vi "Firmware Wizard.vi"() -> ()   [LabVIEW 2011, in "LVH-LINX.lvlib"]
doc: "Wizard for uploading firmware to LINX devices."
uses:
  LVH-LINX.lvlib
  Type Defs/Device Family.ctl
  Type Defs/Deploy Firmware State.ctl
  <vilib>/LabVIEW Hacker/LVH-Toolbox/Common/LVH-Common.lvlib
panel:
  in  "Device Family Enum":T1
  out "Error Out":errorcluster
  in  "Error In":errorcluster
  out "Tab Control":T2(tab)
  in  "Settings Button":bool
  out "Device Image":picture
  in  "Device Help":bool
  in  "Firmware Program Interface":u16(ring) items=["Serial / USB"]
  in  "Device Type":u16(ring) items=["chipKIT Uno32", "chipKIT uC32", "chipKIT Max32", "chipKIT DP32"]
  in  "Device Family":u16(ring) items=["National Instruments", "Digilent", "Arduino"]
  in  "Device Cancel":bool
  in  "Device Next":bool
  in  "Device Noticiation":string
  in  "Config Message":string
  in  "Int Help":bool
  in  "Int Previous":bool
  in  "Int Cancel":bool
  in  "Int Next":bool
  out "Interface Config":enum32{"N/A", "Serial / USB", "USB", "TCP"}(tab)
  in  "COM Port":refnum<visa-resource-name>
  in  "Firmware Description":string
  in  "FWV Help":bool
  in  "FWV Cancel":bool
  in  "FWV Next":bool
  in  "FWV Previous":bool
  in  "Firmware Version":u16(ring) items=["LINX -  Serial / USB", "LINX -  Serial / USB [Debug] "]
  in  "Deploy  Progress Bar":u8(slide) scale=0.0..100.0
  in  "LINX Forum Link":string="www.labviewhacker.com/forums/linx"
  in  "LINX Landing Page Link":string="www.labviewhacker.com/linx"
  in  "Summary Launch Example":bool
  in  "Summary Text":string
  in  "Summary Next":bool
  in  "Summary Help":bool
  # "Uploading Firmware..."
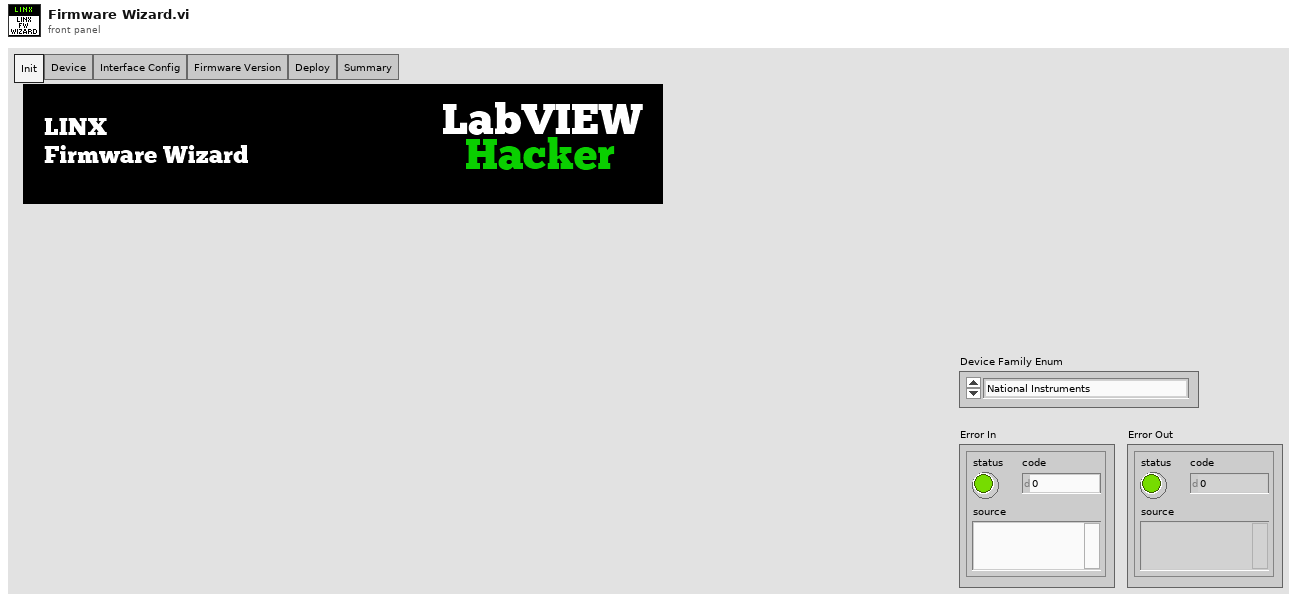
[diagram p1: front panel]
types:
  T1 = typedef "LVH-LINX.lvlib/Device Family.ctl" = enum8{"National Instruments", "Digilent", "Arduino"}
  T2 = enum32{"Init", "Device", "Interface Config", "Firmware Version", "Deploy", "Summary"}
  T3 = typedef "LVH-LINX.lvlib/Deploy Firmware State.ctl" = enum32{"Init", "Device", "Interface Config", "Firmware Version", "Deploy", "Summary"}
  T4 = enum16{"Left Button", "Center Button", "Right Button", "Window Close"}
  T5 = enum32{"invalid app kind", "Development System", "Run Time System", "Student Edition", "Embedded LabVIEW", "Evaluation", "Custom"}
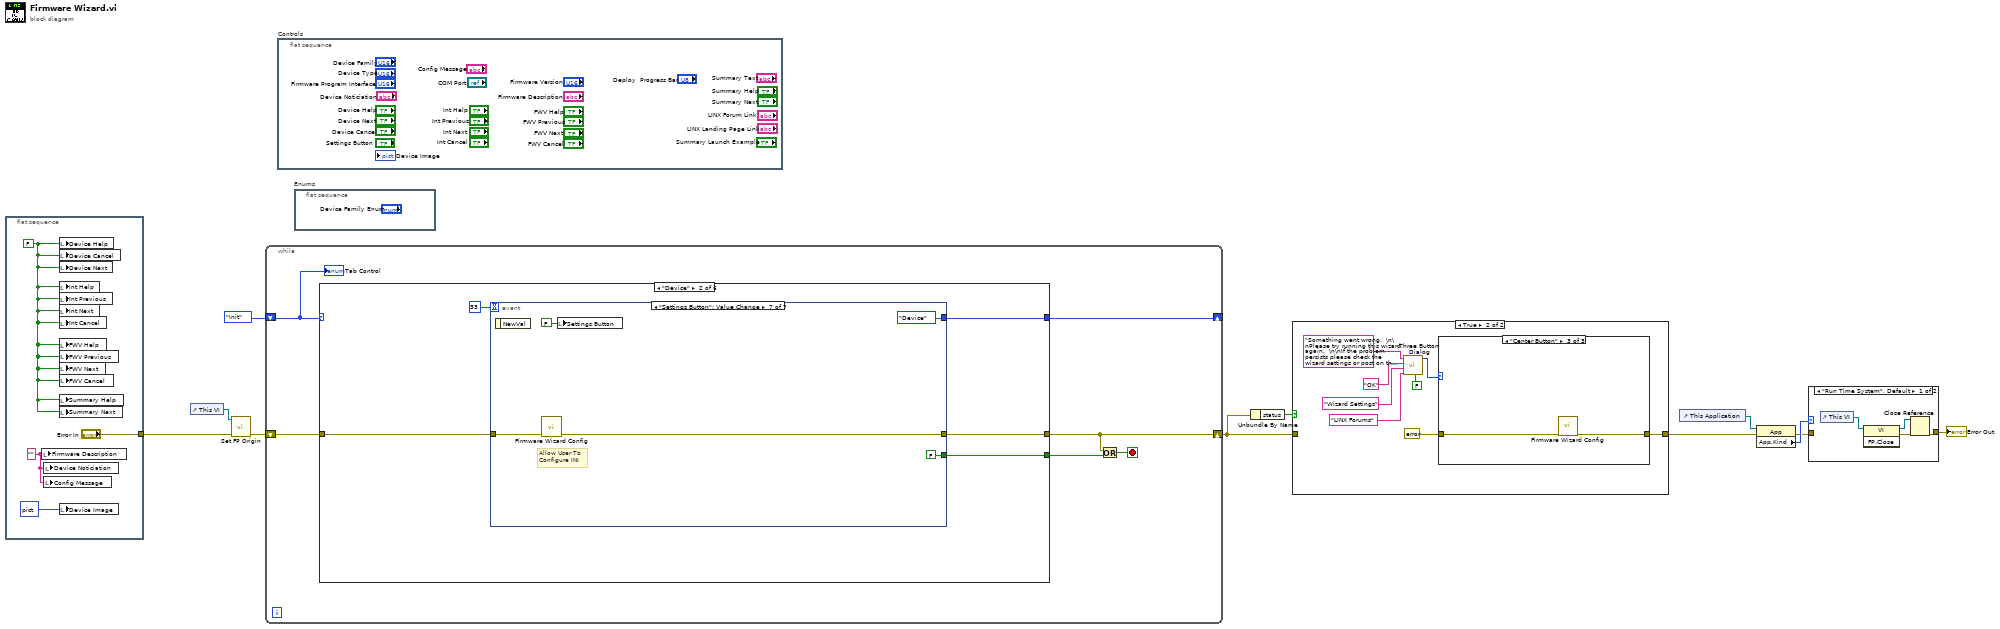
[diagram p0: block diagram]
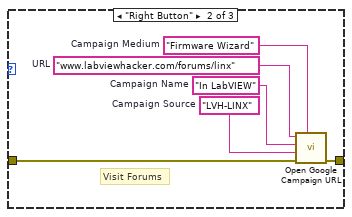
[diagram p4: hidden frame]
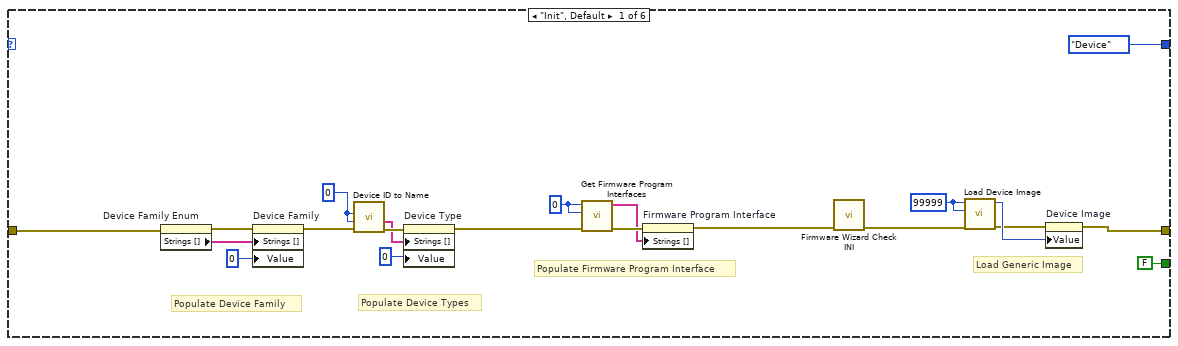
[diagram p6: hidden frame]
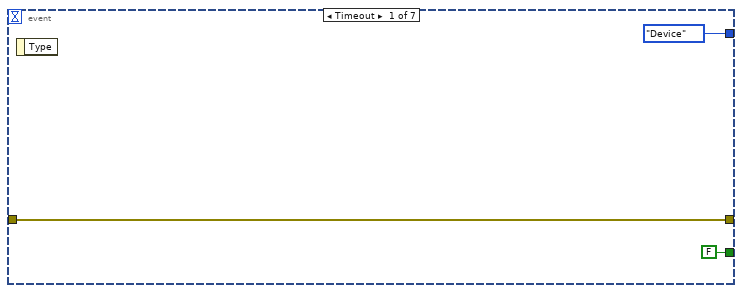
[diagram p7: hidden frame]
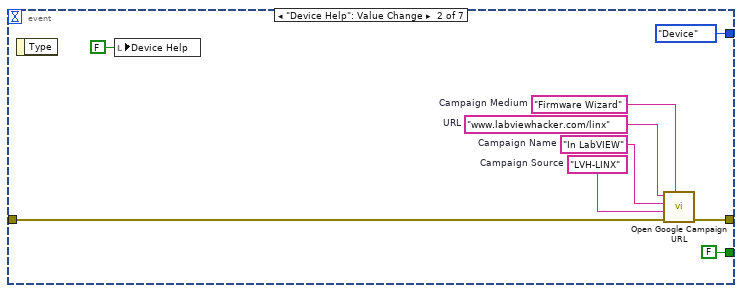
[diagram p8: hidden frame]
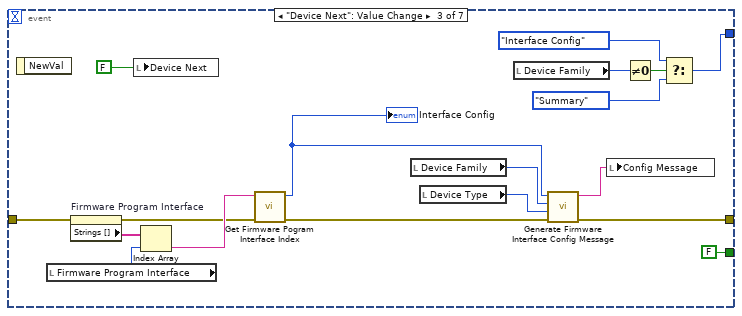
[diagram p9: hidden frame]
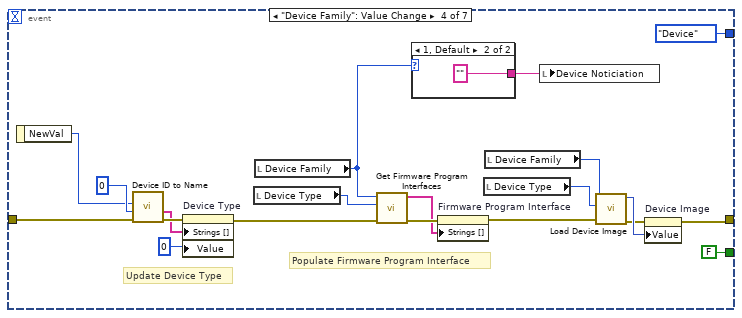
[diagram p10: hidden frame]
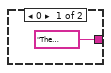
[diagram p11: hidden frame]
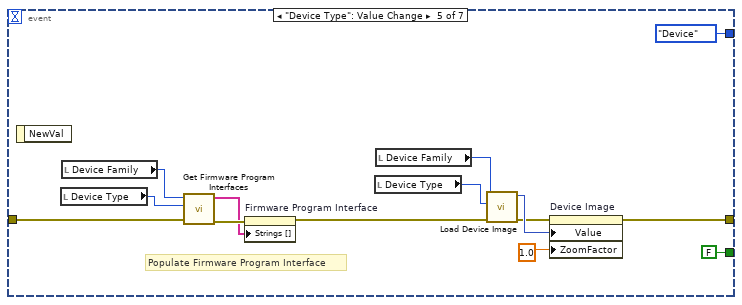
[diagram p12: hidden frame]
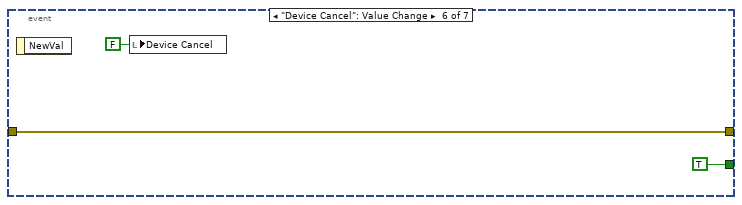
[diagram p13: hidden frame]
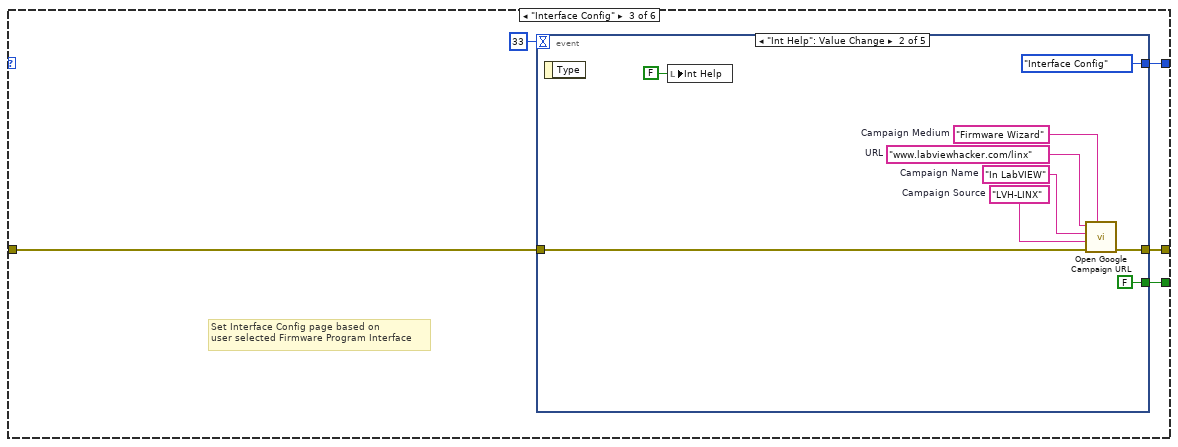
[diagram p14: hidden frame]
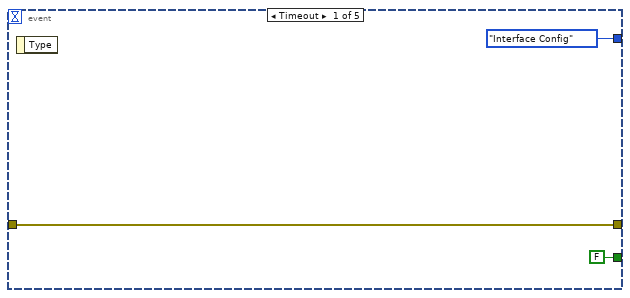
[diagram p15: hidden frame]
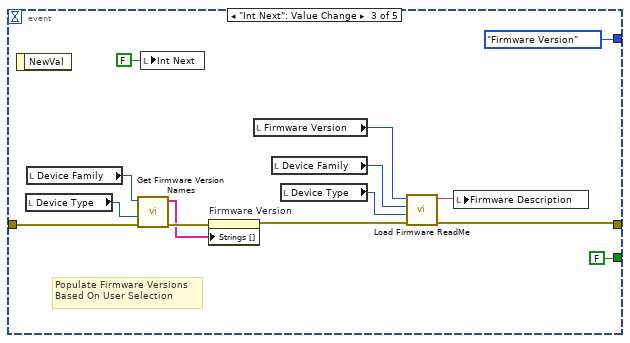
[diagram p16: hidden frame]
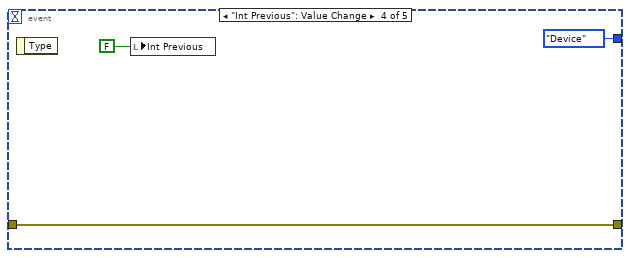
[diagram p17: hidden frame]
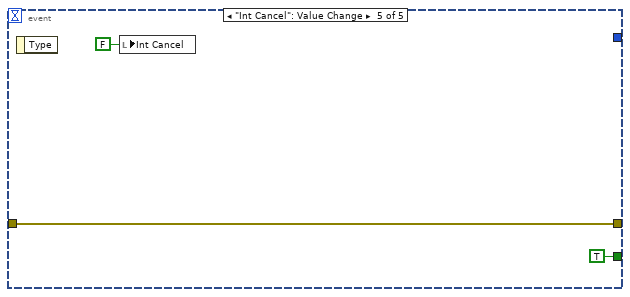
[diagram p18: hidden frame]
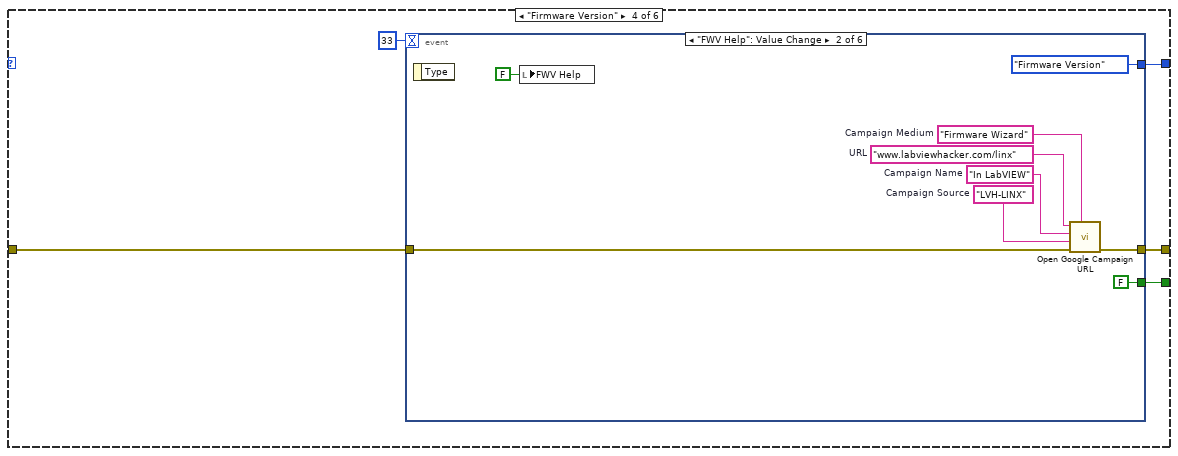
[diagram p19: hidden frame]
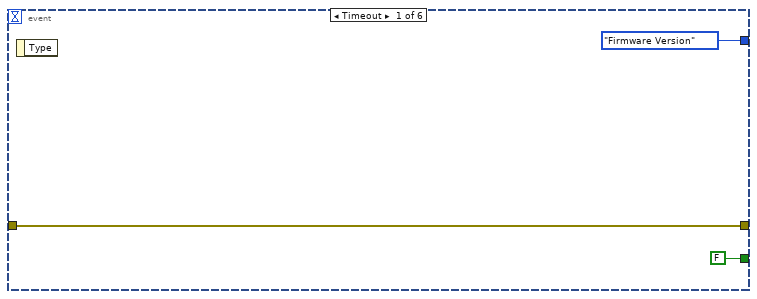
[diagram p20: hidden frame]
diagram:
  n1 = flat-sequence {
    tunnel: ["Error In"] -> w9
    frame #0 {
      w12 = "" ("Firmware Description")
      w14 = FALSE ("Cancel")
      n2 = local write "Firmware Description"(w12) -> ()
      n3 = local write "Device Noticiation"(w12) -> ()
      n4 = local write "Config Message"(w12) -> ()
      n5 = local write "Device Help"(w14) -> ()
      n6 = local write "Device Cancel"(w14) -> ()
      n7 = local write "Device Next"(w14) -> ()
      n8 = local write "Int Help"(w14) -> ()
      n9 = local write "Int Previous"(w14) -> ()
      n10 = local write "Int Next"(w14) -> ()
      n11 = local write "Int Cancel"(w14) -> ()
      n12 = local write "FWV Help"(w14) -> ()
      n13 = local write "FWV Previous"(w14) -> ()
      n14 = local write "FWV Next"(w14) -> ()
      n15 = local write "FWV Cancel"(w14) -> ()
      n16 = local write "Summary Help"(w14) -> ()
      n17 = local write "Summary Next"(w14) -> ()
      n18 = local write "Device Image"(picture data[5B] ("2D Picture")) -> ()
    }
  }
  n19 = control-ref of="This VI"() -> (w10:refnum<vi>)
  n20 = call <vilib>:"Set FP Origin.vi"("Error In"=w9, "VI Ref"=w10) -> ("Error Out"=w8:errorcluster)  [unwired: 9 in]
  n21 = while {
    shift-right: [w19] -> _
    shift-left: Deploy_Firmware_State."Init" ("Deploy Firmware State") -> [w21]
    shift-right: [w18] -> w1
    shift-left: w8 -> [w20]
    stop <- w17 stop-if-true
    n22 = case shown="\"Device\"" w21 {
      tunnel: [w25 w46 w125 w163 w201 w213] -> w18
      tunnel: w20 -> [w29 w45 w122 w162 w202 w209]
      tunnel: [Deploy_Firmware_State."Device" ("Deploy Firmware State") w44 w126 w160 Deploy_Firmware_State."Summary" ("Deploy Firmware State") w211] -> w19
      tunnel: [FALSE w43 w123 w159 FALSE w210] -> w16
      frame "Init", Default {
        w24 = u32 99999 ("Device Family")
        w30 = u32 0 ("Device Family")
        w36 = u32 0 ("Device Family")
        # "Load Generic Image"
        # "Populate Firmware Program Interface"
        # "Populate Device Types"
        # "Populate Device Family"
        n23 = property on="Device Family Enum" class="Enum (strict)"(error in=w29) -> (error out=w41:errorcluster, "Strings []"=w40:string[])  [unwired: 1 in, 1 out]
        n24 = property on="Device Family" class="Ring (strict)"(error in=w41, "Strings []"=w40, "Value"=u16 0 ("Device Family")) -> (error out=w38:errorcluster)  [unwired: 1 in, 1 out]
        n25 = call "Device ID to Name.vi"("Error In"=w38, "Device ID"=w36, "Device Family"=w36) -> ("Error Out"=w37:errorcluster, "Devices In Family"=w35:string[])  [unwired: 5 in, 2 out]
        n26 = property on="Device Type" class="Ring (strict)"(error in=w37, "Strings []"=w35, "Value"=u16 0 ("Device Family")) -> (error out=w31:errorcluster)  [unwired: 1 in, 1 out]
        n27 = call "Get Firmware Program Interfaces.vi"("Error In"=w31, "Device ID"=w30, "Device Family"=w30) -> ("Error Out"=w33:errorcluster, "Firmware Program Interfaces"=w32:string[])  [unwired: 7 in]
        n28 = property on="Firmware Program Interface" class="Ring (strict)"(error in=w33, "Strings []"=w32) -> (error out=w23:errorcluster)  [unwired: 1 in, 1 out]
        n29 = call "Firmware Wizard Check INI.vi"("Error In"=w23) -> ("Error Out"=w22:errorcluster)  [unwired: 10 in]
        n30 = call "Load Device Image.vi"("Error In"=w22, "Device Type"=w24, "Device Family"=w24) -> ("Error Out"=w26:errorcluster, "Device Image"=w27:picture)  [unwired: 7 in]
        n31 = property on="Device Image" class="Pict"(error in=w26, "Value"=w27) -> (error out=w25:errorcluster)  [unwired: 1 in, 1 out]
      }
      frame "Device" {
        n32 = event shown="[6] \"Settings Button\": Value Change" {
          selector: _ -> [_ _ _ _ _ _ _]
          dyn-events: _ -> [_ _ _ _ _ _ _]
          timeout: 33 -> [_ _ _ _ _ _ _]
          tunnel: [w50 w53 w68 w80 w100 w115 w118] -> w46
          tunnel: w45 -> [w50 w52 w62 w93 w113 w115 w119]
          tunnel: [Deploy_Firmware_State."Device" ("Deploy Firmware State") Deploy_Firmware_State."Device" ("Deploy Firmware State") w71 Deploy_Firmware_State."Device" ("Deploy Firmware State") Deploy_Firmware_State."Device" ("Deploy Firmware State") _ Deploy_Firmware_State."Device" ("Deploy Firmware State")] -> w44
          tunnel: [FALSE FALSE FALSE FALSE FALSE TRUE FALSE] -> w43
          event Timeout {
            n33 = event-data() -> ()  [unwired: 1 in, 1 out]
          }
          event "Device Help": Value Change {
            w51 = "LVH-LINX"  # Campaign Source
            w54 = "In LabVIEW"  # Campaign Name
            w55 = "Firmware Wizard"  # Campaign Medium
            w56 = "www.labviewhacker.com/linx"  # URL
            n34 = event-data() -> ()  [unwired: 1 in, 1 out]
            n35 = local write "Device Help"(FALSE ("Device Help")) -> ()
            n36 = call <vilib>:"Open Google Campaign URL.vi"("Campaign Medium"=w55, "Error In"=w52, "Campaign Source"=w51, "Campaign Name"=w54, "URL"=w56) -> ("Error Out"=w53:errorcluster)  [unwired: 5 in, 1 out]
          }
          event "Device Next": Value Change {
            n37 = event-data() -> ()  [unwired: 1 in, 1 out]
            n38 = local read "Firmware Program Interface"() -> (w63:u16)
            n39 = property on="Firmware Program Interface" class="Ring (strict)"(error in=w62) -> (error out=w64:errorcluster, "Strings []"=w66:string[])  [unwired: 1 in, 1 out]
            n40 = local write "Device Next"(FALSE ("Next")) -> ()
            n41 = Index Array(array=w66, index=w63) -> (element=w65:string)
            n42 = call "Get Firmware Pogram Interface Index.vi"("Error In"=w64, "Firmware Program Interface"=w65) -> ("Error Out"=w61:errorcluster, "Interface Index"=w60:i32)  [unwired: 8 in]
            "Interface Config" <- w60
            n43 = local read "Device Family"() -> (w70:u16)
            n44 = local read "Device Type"() -> (w67:u16)
            n45 = local read "Device Family"() -> (w74:u16)
            n46 = call "Generate Firmware Interface Config Message.vi"("Error In"=w61, "Device Type"=w67, "Device Family"=w70, "Firmware Program Interface"=w60) -> ("Error Out"=w68:errorcluster, "Config Message"=w69:string)  [unwired: 6 in]
            n47 = local write "Config Message"(w69) -> ()
            n48 = Not Equal To 0?(x=w74) -> (x != 0?=w75:bool)
            n49 = Select(t=Deploy_Firmware_State."Interface Config" ("Deploy Firmware State"), s=w75, f=Deploy_Firmware_State."Summary" ("Deploy Firmware State")) -> (s? t:f=w71:T3)
          }
          event "Device Family": Value Change {
            # "Populate Firmware Program Interface"
            # "Update Device Type"
            n50 = event-data() -> ("NewVal"=w92:u16)  [unwired: 1 in]
            n51 = call "Device ID to Name.vi"("Error In"=w93, "Device ID"=u32 0 ("Device Family"), "Device Family"=w92) -> ("Error Out"=w97:errorcluster, "Devices In Family"=w95:string[])  [unwired: 5 in, 2 out]
            n52 = property on="Device Type" class="Ring (strict)"(error in=w97, "Strings []"=w95, "Value"=u16 0 ("Device Family")) -> (error out=w87:errorcluster)  [unwired: 1 in, 1 out]
            n53 = local read "Device Type"() -> (w88:u16)
            n54 = local read "Device Family"() -> (w79:u16)
            n55 = call "Get Firmware Program Interfaces.vi"("Error In"=w87, "Device ID"=w88, "Device Family"=w79) -> ("Error Out"=w90:errorcluster, "Firmware Program Interfaces"=w89:string[])  [unwired: 7 in]
            n56 = case shown="1, Default" w79 {
              tunnel: ["The National Instruments devices that support LINX do not require firmware updates." ("Device Noticiation") "" ("Device Noticiation")] -> w78
              frame 0 {
              }
              frame 1, Default {
              }
            }
            n57 = property on="Firmware Program Interface" class="Ring (strict)"(error in=w90, "Strings []"=w89) -> (error out=w81:errorcluster)  [unwired: 1 in, 1 out]
            n58 = local read "Device Type"() -> (w85:u16)
            n59 = local read "Device Family"() -> (w84:u16)
            n60 = local write "Device Noticiation"(w78) -> ()
            n61 = call "Load Device Image.vi"("Error In"=w81, "Device Type"=w85, "Device Family"=w84) -> ("Error Out"=w82:errorcluster, "Device Image"=w83:picture)  [unwired: 7 in]
            n62 = property on="Device Image" class="Pict"(error in=w82, "Value"=w83) -> (error out=w80:errorcluster)  [unwired: 1 in, 1 out]
          }
          event "Device Type": Value Change {
            # "Populate Firmware Program Interface"
            n63 = event-data() -> ()  [unwired: 1 in, 1 out]
            n64 = local read "Device Type"() -> (w109:u16)
            n65 = local read "Device Family"() -> (w108:u16)
            n66 = call "Get Firmware Program Interfaces.vi"("Error In"=w113, "Device ID"=w109, "Device Family"=w108) -> ("Error Out"=w112:errorcluster, "Firmware Program Interfaces"=w111:string[])  [unwired: 7 in]
            n67 = property on="Firmware Program Interface" class="Ring (strict)"(error in=w112, "Strings []"=w111) -> (error out=w106:errorcluster)  [unwired: 1 in, 1 out]
            n68 = local read "Device Type"() -> (w105:u16)
            n69 = local read "Device Family"() -> (w104:u16)
            n70 = call "Load Device Image.vi"("Error In"=w106, "Device Type"=w105, "Device Family"=w104) -> ("Error Out"=w101:errorcluster, "Device Image"=w103:picture)  [unwired: 7 in]
            n71 = property on="Device Image" class="Pict"(error in=w101, "Value"=w103, "ZoomFactor"=sgl 1.0 ("Zoom Factor")) -> (error out=w100:errorcluster)  [unwired: 1 in, 1 out]
          }
          event "Device Cancel": Value Change {
            n72 = event-data() -> ()  [unwired: 1 in, 1 out]
            n73 = local write "Device Cancel"(FALSE ("Device Cancel")) -> ()
          }
          event "Settings Button": Value Change {
            # "Allow User To \nConfigure INI"
            n74 = event-data() -> ()  [unwired: 1 in, 1 out]
            n75 = call "Firmware Wizard Config.vi"("Error In"=w119) -> ("Error Out"=w118:errorcluster)  [unwired: 10 in]
            n76 = local write "Settings Button"(FALSE ("Settings Button")) -> ()
          }
        }
      }
      frame "Interface Config" {
        # "Set Interface Config page based on \nuser selected Firmware Program Interface"
        n77 = event shown="[1] \"Int Help\": Value Change" {
          selector: _ -> [_ _ _ _ _]
          dyn-events: _ -> [_ _ _ _ _]
          timeout: 33 -> [_ _ _ _ _]
          tunnel: [Deploy_Firmware_State."Interface Config" ("Deploy Firmware State") Deploy_Firmware_State."Interface Config" ("Deploy Firmware State") Deploy_Firmware_State."Firmware Version" ("Deploy Firmware State") Deploy_Firmware_State."Device" ("Deploy Firmware State") _] -> w126
          tunnel: [w128 w130 w139 w155 w156] -> w125
          tunnel: w122 -> [w128 w131 w152 w155 w156]
          tunnel: [FALSE FALSE FALSE _ TRUE] -> w123
          event Timeout {
            n78 = event-data() -> ()  [unwired: 1 in, 1 out]
          }
          event "Int Help": Value Change {
            w132 = "LVH-LINX"  # Campaign Source
            w133 = "In LabVIEW"  # Campaign Name
            w134 = "Firmware Wizard"  # Campaign Medium
            w135 = "www.labviewhacker.com/linx"  # URL
            n79 = event-data() -> ()  [unwired: 1 in, 1 out]
            n80 = local write "Int Help"(FALSE ("Int Help")) -> ()
            n81 = call <vilib>:"Open Google Campaign URL.vi"("Campaign Medium"=w134, "Error In"=w131, "Campaign Source"=w132, "Campaign Name"=w133, "URL"=w135) -> ("Error Out"=w130:errorcluster)  [unwired: 5 in, 1 out]
          }
          event "Int Next": Value Change {
            # "Populate Firmware Versions\nBased On User Selection"
            n82 = event-data() -> ()  [unwired: 1 in, 1 out]
            n83 = local read "Device Type"() -> (w149:u16)
            n84 = local read "Device Family"() -> (w148:u16)
            n85 = call "Get Firmware Version Names.vi"("Error In"=w152, "Device ID"=w149, "Device Family"=w148) -> ("Error Out"=w151:errorcluster, "Firmware Version Names"=w150:string[])  [unwired: 6 in, 1 out]
            n86 = local write "Int Next"(FALSE ("Int Next")) -> ()
            n87 = property on="Firmware Version" class="Ring (strict)"(error in=w151, "Strings []"=w150) -> (error out=w140:errorcluster)  [unwired: 1 in, 1 out]
            n88 = local read "Firmware Version"() -> (w142:u16)
            n89 = local read "Device Family"() -> (w144:u16)
            n90 = local read "Device Type"() -> (w143:u16)
            n91 = call "Load Firmware ReadMe.vi"("Error In"=w140, "Device Family"=w143, "Device Type"=w144, "Firmware Version"=w142) -> ("Error Out"=w139:errorcluster, "Firmware ReadMe"=w141:string)  [unwired: 6 in]
            n92 = local write "Firmware Description"(w141) -> ()
          }
          event "Int Previous": Value Change {
            n93 = event-data() -> ()  [unwired: 1 in, 1 out]
            n94 = local write "Int Previous"(FALSE ("Previous")) -> ()
          }
          event "Int Cancel": Value Change {
            n95 = event-data() -> ()  [unwired: 1 in, 1 out]
            n96 = local write "Int Cancel"(FALSE ("Int Cancel")) -> ()
          }
        }
      }
      frame "Firmware Version" {
        n97 = event shown="[1] \"FWV Help\": Value Change" {
          selector: _ -> [_ _ _ _ _ _]
          dyn-events: _ -> [_ _ _ _ _ _]
          timeout: 33 -> [_ _ _ _ _ _]
          tunnel: [w166 w168 w178 w182 w186 w192] -> w163
          tunnel: w162 -> [w166 w167 w178 w182 w186 w193]
          tunnel: [Deploy_Firmware_State."Firmware Version" ("Deploy Firmware State") Deploy_Firmware_State."Firmware Version" ("Deploy Firmware State") Deploy_Firmware_State."Interface Config" ("Deploy Firmware State") Deploy_Firmware_State."Deploy" ("Deploy Firmware State") Deploy_Firmware_State."Init" ("Deploy Firmware State") Deploy_Firmware_State."Firmware Version" ("Deploy Firmware State")] -> w160
          tunnel: [FALSE FALSE FALSE FALSE TRUE FALSE] -> w159
          event Timeout {
            n98 = event-data() -> ()  [unwired: 1 in, 1 out]
          }
          event "FWV Help": Value Change {
            w169 = "LVH-LINX"  # Campaign Source
            w170 = "In LabVIEW"  # Campaign Name
            w171 = "Firmware Wizard"  # Campaign Medium
            w172 = "www.labviewhacker.com/linx"  # URL
            n99 = event-data() -> ()  [unwired: 1 in, 1 out]
            n100 = local write "FWV Help"(FALSE ("FWV Help")) -> ()
            n101 = call <vilib>:"Open Google Campaign URL.vi"("Campaign Medium"=w171, "Error In"=w167, "Campaign Source"=w169, "Campaign Name"=w170, "URL"=w172) -> ("Error Out"=w168:errorcluster)  [unwired: 5 in, 1 out]
          }
          event "FWV Previous": Value Change {
            n102 = event-data() -> ()  [unwired: 1 in, 1 out]
            n103 = local write "FWV Previous"(FALSE ("FWV Previous")) -> ()
          }
          event "FWV Next": Value Change {
            n104 = event-data() -> ()  [unwired: 1 in, 1 out]
            n105 = local write "FWV Next"(FALSE ("FWV Previous")) -> ()
          }
          event "FWV Cancel": Value Change {
            n106 = event-data() -> ()  [unwired: 1 in, 1 out]
            n107 = local write "FWV Cancel"(FALSE ("FWV Previous")) -> ()
          }
          event "Firmware Version": Value Change {
            n108 = event-data() -> ()  [unwired: 1 in, 1 out]
            n109 = local read "Firmware Version"() -> (w189:u16)
            n110 = local read "Device Family"() -> (w191:u16)
            n111 = local read "Device Type"() -> (w190:u16)
            n112 = call "Load Firmware ReadMe.vi"("Error In"=w193, "Device Family"=w190, "Device Type"=w191, "Firmware Version"=w189) -> ("Error Out"=w192:errorcluster, "Firmware ReadMe"=w188:string)  [unwired: 6 in]
            n113 = local write "Firmware Description"(w188) -> ()
          }
        }
      }
      frame "Deploy" {
        n114 = control-ref of="Deploy  Progress Bar"() -> (w196:refnum<vi>)
        n115 = local read "Firmware Version"() -> (w200:u16)
        n116 = local read "Device Family"() -> (w198:u16)
        n117 = local read "Device Type"() -> (w199:u16)
        n118 = local read "COM Port"() -> (w197:refnum<visa-resource-name>)
        n119 = call "Upload Firmware.vi"("Progress Bar"=w196, "COM Port"=w197, "Error In"=w202, "Firmware Version"=w200, "Device ID"=w199, "Device Family"=w198) -> ("Error Out"=w201:errorcluster)  [unwired: 5 in]
      }
      frame "Summary" {
        n120 = local read "Device Family"() -> (w207:u16)
        n121 = local read "Device Type"() -> (w206:u16)
        n122 = call "Generate Firmware Wizard Summary Message.vi"("Error In"=w209, "Device ID"=w206, "Device Family"=w207) -> ("Error Out"=w208:errorcluster, "Summary"=w205:string)  [unwired: 7 in]
        n123 = local write "Summary Text"(w205) -> ()
        n124 = event shown="[3] \"Summary Help\": Value Change" {
          selector: _ -> [_ _ _ _ _ _]
          dyn-events: _ -> [_ _ _ _ _ _]
          timeout: 33 -> [_ _ _ _ _ _]
          tunnel: [w216 w223 w230 w238 w240 w245] -> w213
          tunnel: w208 -> [w216 w222 w229 w237 w240 w245]
          tunnel: [Deploy_Firmware_State."Summary" ("Deploy Firmware State") Deploy_Firmware_State."Summary" ("Deploy Firmware State") Deploy_Firmware_State."Summary" ("Deploy Firmware State") Deploy_Firmware_State."Summary" ("Deploy Firmware State") Deploy_Firmware_State."Summary" ("Deploy Firmware State") Deploy_Firmware_State."Init" ("Deploy Firmware State")] -> w211
          tunnel: [FALSE _ _ _ _ TRUE] -> w210
          event Timeout {
            n125 = event-data() -> ()  [unwired: 1 in, 1 out]
          }
          event "LINX Forum Link": Mouse Down {
            w218 = "LVH-LINX"  # Campaign Source
            w219 = "In LabVIEW"  # Campaign Name
            w220 = "Firmware Wizard"  # Campaign Medium
            w221 = "www.labviewhacker.com/forum/linx"  # URL
            n126 = event-data() -> ()  [unwired: 1 in, 7 out]
            n127 = call <vilib>:"Open Google Campaign URL.vi"("Campaign Medium"=w220, "Error In"=w222, "Campaign Source"=w218, "Campaign Name"=w219, "URL"=w221) -> ("Error Out"=w223:errorcluster)  [unwired: 5 in, 1 out]
          }
          event "LINX Landing Page Link": Mouse Down {
            w225 = "LVH-LINX"  # Campaign Source
            w226 = "In LabVIEW"  # Campaign Name
            w227 = "Firmware Wizard"  # Campaign Medium
            w228 = "www.labviewhacker.com/linx"  # URL
            n128 = event-data() -> ()  [unwired: 1 in, 7 out]
            n129 = call <vilib>:"Open Google Campaign URL.vi"("Campaign Medium"=w227, "Error In"=w229, "Campaign Source"=w225, "Campaign Name"=w226, "URL"=w228) -> ("Error Out"=w230:errorcluster)  [unwired: 5 in, 1 out]
          }
          event "Summary Help": Value Change {
            w233 = "LVH-LINX"  # Campaign Source
            w234 = "In LabVIEW"  # Campaign Name
            w235 = "Firmware Wizard"  # Campaign Medium
            w236 = "www.labviewhacker.com/linx"  # URL
            n130 = event-data() -> ()  [unwired: 1 in, 1 out]
            n131 = local write "Summary Help"(FALSE ("Summary Help")) -> ()
            n132 = call <vilib>:"Open Google Campaign URL.vi"("Campaign Medium"=w235, "Error In"=w237, "Campaign Source"=w233, "Campaign Name"=w234, "URL"=w236) -> ("Error Out"=w238:errorcluster)  [unwired: 5 in, 1 out]
          }
          event "Summary Launch Example": Value Change {
            n133 = event-data() -> ()  [unwired: 1 in, 1 out]
            n134 = local write "Summary Launch Example"(FALSE ("Summary Launch Example")) -> ()
            n135 = One Button Dialog(message="Feature Not Yet Implemented") -> ()  [unwired: 1 in, 1 out]
          }
          event "Summary Next": Value Change {
            n136 = event-data() -> ()  [unwired: 1 in, 1 out]
            n137 = local write "Summary Next"(FALSE ("FWV Previous")) -> ()
          }
        }
      }
    }
    n138 = Or(x=w18, y=w16) -> (x .or. y?=w17:bool)
    "Tab Control" <- w21
  }
  n139 = flat-sequence "Controls" {
    frame #0 {
    }
  }
  n140 = flat-sequence "Enums" {
    frame #0 {
    }
  }
  n141 = Unbundle By Name(w1) -> ("status"=w3:bool)
  n142 = case shown="True" w3 {
    tunnel: [w247 w254] -> w2
    tunnel: w1 -> [w247 _]
    frame False {
    }
    frame True {
      n143 = call <vilib>:"Three Button Dialog.vi"("Allow user to close window? (TRUE)"=FALSE, "Right Button Text (\"Cancel\")"="LINX Forums" ("F button name (\"Cancel\")"), "Center Button Text (\"No\")"="Wizard Settings" ("F button name (\"Cancel\")"), "Left Button Text (\"Yes\")"="OK" ("Left Button Text (\"Yes\")"), "message"="Something went wrong.  \n\nPlease try running this wizard again.  \n\nIf the problem persists please check the wizard settings or post on the LVH LINX Forums at: \n\nwww.labviewhacker.com/forums/linx ") -> ("Which Button?"=w249:T4)  [unwired: 6 in]
      n144 = case shown="\"Center Button\"" w249 {
        tunnel: errorcluster {"status"=FALSE, "code"=0, "source"=""} ("error constant") -> [w256 w258 w264]
        tunnel: [w256 w257 w263] -> w254
        frame "Left Button", Default {
          # "Nothing To Do Here"
        }
        frame "Right Button" {
          w259 = "LVH-LINX"  # Campaign Source
          w260 = "In LabVIEW"  # Campaign Name
          w261 = "Firmware Wizard"  # Campaign Medium
          w262 = "www.labviewhacker.com/forums/linx"  # URL
          # "Visit Forums"
          n145 = call <vilib>:"Open Google Campaign URL.vi"("Campaign Medium"=w261, "Error In"=w258, "Campaign Source"=w259, "Campaign Name"=w260, "URL"=w262) -> ("Error Out"=w257:errorcluster)  [unwired: 5 in, 1 out]
        }
        frame "Center Button" {
          n146 = call "Firmware Wizard Config.vi"("Error In"=w264) -> ("Error Out"=w263:errorcluster)  [unwired: 10 in]
        }
      }
    }
  }
  n147 = control-ref of="This Application"() -> (w6:refnum<vi>)
  n148 = property class="App"(reference=w6, error in=w2) -> (error out=w4:errorcluster, "App.Kind"=w5:T5)  [unwired: 1 out]
  n149 = case shown="\"Run Time System\", Default" w5 {
    tunnel: [w266 w269] -> w7
    tunnel: w4 -> [_ w269]
    frame "Run Time System", Default {
      n150 = control-ref of="This VI"() -> (w265:refnum<vi>)
      n151 = invoke class="VI" method="FP.Close"(reference=w265) -> (reference out=w268:refnum<vi>, error out=w267:errorcluster)  [unwired: 2 in, 1 out]
      n152 = Close Reference(reference=w268, error in (no error)=w267) -> (error out=w266:errorcluster)
    }
    frame "Development System" {
    }
  }
  "Error Out" <- w7
